vi "feedback-positive.vi"(7 "callee":refnum<vi>, 8 "error in (no error)":errorcluster, 10 "process_error":errorcluster, 11 "dialog_text":string) -> (0 "error out":errorcluster)   [LabVIEW 2015, in "lv-dialog.lvlib"]
uses:
  api/v1/public/class/v1.lvclass
  lv-dialog.lvlib
  api/v1/v1.lvlib
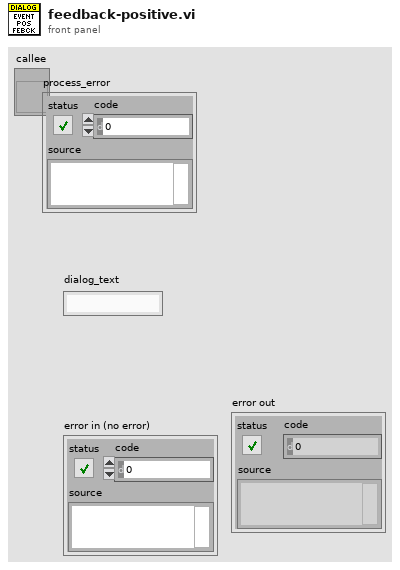
[diagram p1: front panel]
types:
  T1 = cluster{"dialog_text":string, "boolean_text_1":string}
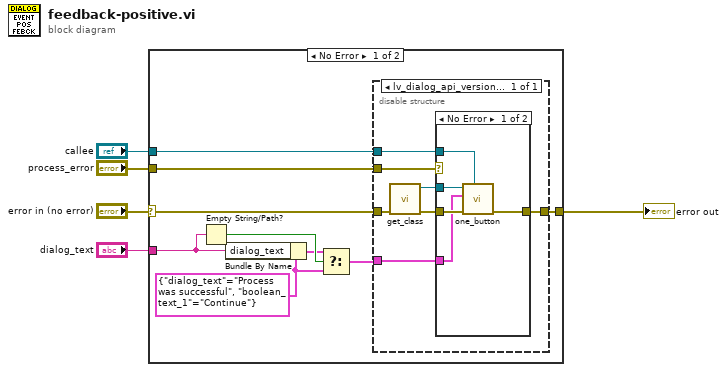
[diagram p0: block diagram]
diagram:
  n1 = case shown="No Error" "error in (no error)" {
    selector: "error in (no error)" -> [w9 w28]
    tunnel: "callee" -> [w14 _]
    tunnel: [w11 w28] -> w1
    tunnel: "process_error" -> [w10 _]
    tunnel: "dialog_text" -> [w8 _]
    frame No Error {
      w6 = T1 {"dialog_text"="Process was successful", "boolean_text_1"="Continue"} ("configuration")
      n2 = Empty String/Path?(string/path=w8) -> (empty?=w13:bool)
      n3 = Bundle By Name(cluster=w6, "dialog_text"=w8) -> (w7:T1)
      n4 = Select(t=w7, s=w13, f=w6) -> (s? t:f=w12:T1)
      n5 = disable-structure shown="lv_dialog_api_version==1, Default" {
        disable-tunnel: w14 -> [w21]
        disable-tunnel: w12 -> [w20]
        disable-tunnel: [w19] -> w11
        disable-tunnel: w10 -> [w18]
        disable-tunnel: w9 -> [w17]
        frame condition #0 (active) {
          n6 = call "get_class.vi"("error in (no error)"=w17) -> ("error out"=w16:errorcluster, "class"=w15:refnum<class "v1.lvclass">)  [unwired: 9 in]
          n7 = case shown="No Error" w18 {
            tunnel: w21 -> [w24 _]
            tunnel: w20 -> [w22 _]
            tunnel: [w26 w27] -> w19
            tunnel: w16 -> [w25 w27]
            tunnel: w15 -> [w23 _]
            frame No Error {
              n8 = call-dynamic "one_button.vi"("callee"=w24, "error in (no error)"=w25, "configuration"=w22, "v1 in"=w23) -> ("error out"=w26:errorcluster)  [unwired: 5 in, 2 out]
            }
            frame Error {
            }
          }
        }
      }
    }
    frame Error {
    }
  }
  "error out" <- w1
